vi "Init UI.vi"(8 "error in (no error)":errorcluster, 11 "Mixer in":refnum<class "Mixer.lvclass">) -> (0 "error out":errorcluster, 3 "Mixer out":refnum<class "Mixer.lvclass">)   [LabVIEW 2019, in "Mixer.lvclass"]
uses:
  Mixer.lvclass
  Packed Libraries/Messaging.lvlibp
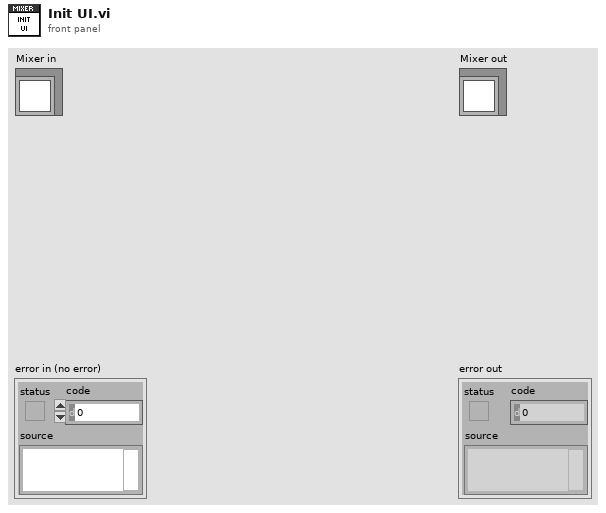
[diagram p1: front panel]
types:
  T1 = typedef "Audio Processing.lvlibp/Value Properties.ctl" = cluster{"Lower":dbl, "Upper":dbl, "Default":dbl, "Increment":dbl}
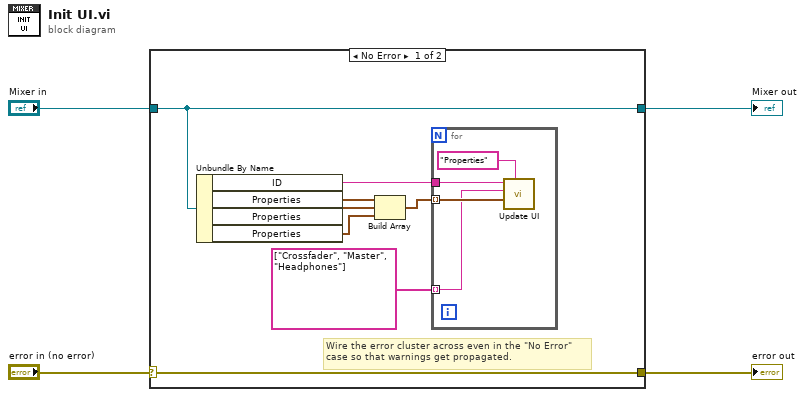
[diagram p0: block diagram]
diagram:
  n1 = case shown="No Error" "error in (no error)" {
    selector: "error in (no error)" -> [w12 w18]
    tunnel: [w12 w18] -> w2
    tunnel: [w11 w17] -> w1
    tunnel: "Mixer in" -> [w11 w17]
    frame No Error {
      # "Wire the error cluster across even in the \"No Error\"\ncase so that warnings get propagated."
      n2 = Unbundle By Name(w11) -> ("ID"=w10:string, "Properties"=w9:T1, "Properties"=w6:T1, "Properties"=w5:T1)
      n3 = Build Array(w9, w6, w5) -> (w8:T1[])
      n4 = for {
        tunnel: w10 -> [w16]
        tunnel: w8 -> [w15] mode=indexing
        tunnel: string[] ["Crossfader", "Master", "Headphones"] -> [w14] mode=indexing
        n5 = call "Update UI.vi"("Message (Value Change)"="Properties", "Data"=w15, "Target"=w14, "ID"=w16) -> ()  [unwired: 7 in, 1 out]
      }
    }
    frame Error {
    }
  }
  "error out" <- w2
  "Mixer out" <- w1
